vi "WaitForConnection.vi"(8 "error in (no error)":errorcluster, 11 "Tcp in":refnum<class "Tcp.lvclass">) -> (0 "error out":errorcluster, 3 "Tcp out":refnum<class "Tcp.lvclass">)   [LabVIEW 2022 SP3, in "Tcp.lvlib" / "Tcp.lvclass"]
uses:
  Tcp.lvclass
  Tcp.lvclass/Tcp.ctl
  <vilib>/ActorFramework/Actor/Actor.lvclass
  Connection/Connection/Connection.lvclass
  Connection/Connection Messages/Initialize Msg/Initialize Msg.lvclass
  C:/Program Files (x86)/National Instruments/LabVIEW 2022/vi.lib/ActorFramework/Actor/Actor.lvclass
  Tcp Messages/WaitForConnection Msg/WaitForConnection Msg.lvclass
  TcpSocket/Source/TcpSocket/TcpServer/TcpServer.lvclass
  TcpSocket/Source/TcpSocket/Connection/Connection.lvclass
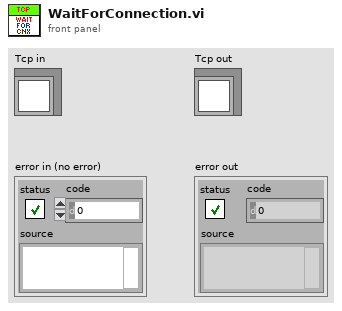
[diagram p1: front panel]
types:
  T1 = map{u64, refnum<class "Message Enqueuer.lvclass">}
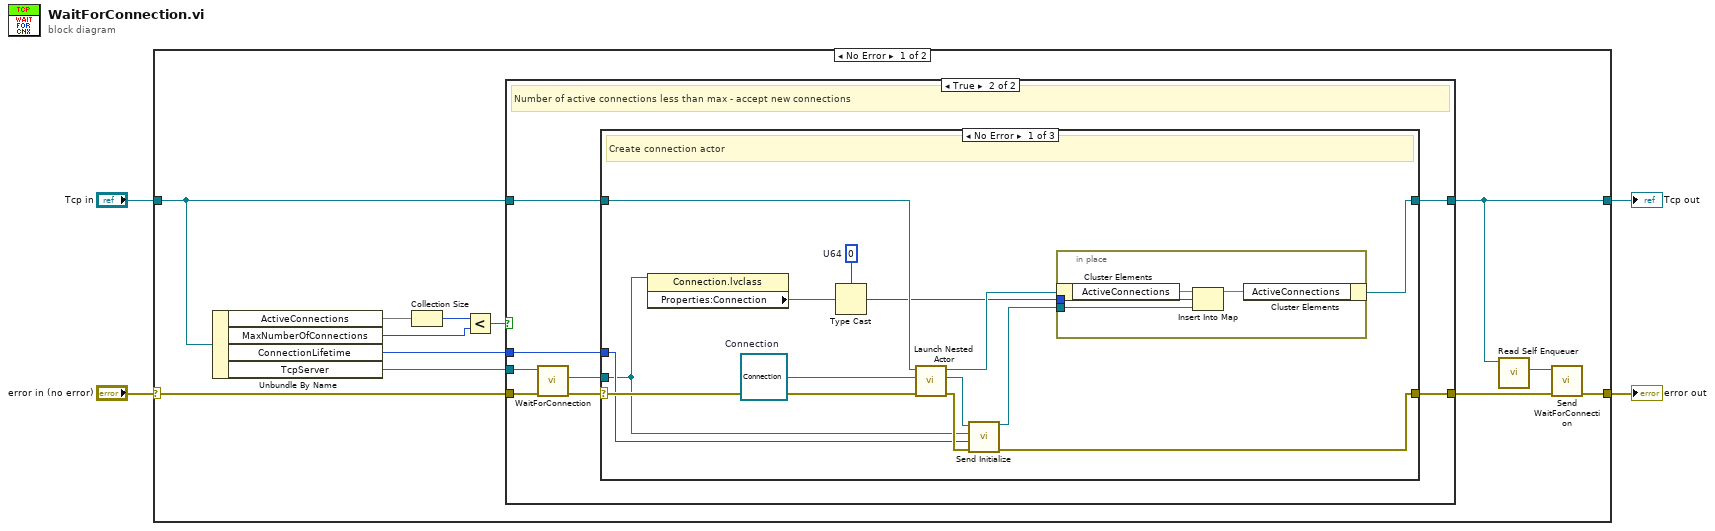
[diagram p0: block diagram]
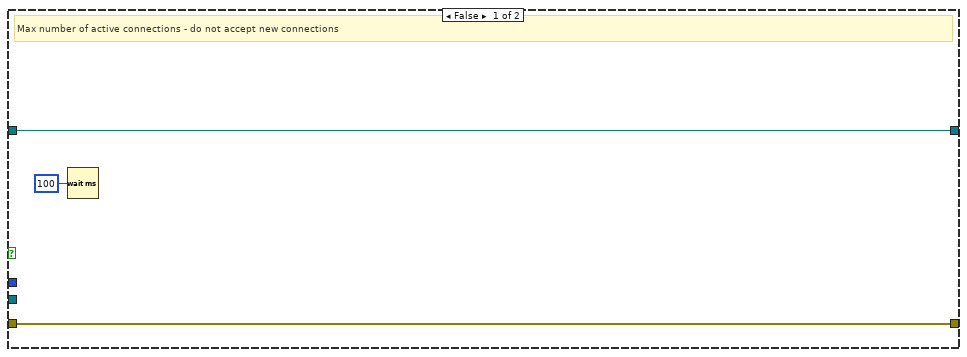
[diagram p2: hidden frame]
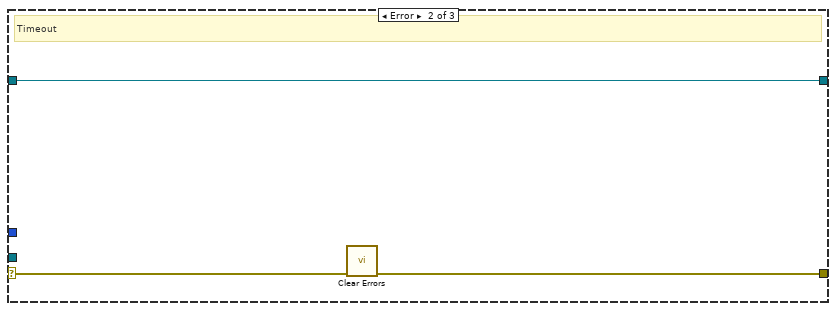
[diagram p3: hidden frame]
diagram:
  n1 = case shown="No Error" "error in (no error)" {
    selector: "error in (no error)" -> [w16 w52]
    tunnel: [w10 w52] -> w3
    tunnel: [w12 w51] -> w1
    tunnel: "Tcp in" -> [w14 w51]
    frame No Error {
      n2 = Unbundle By Name(w14) -> ("ActiveConnections"=w8:T1, "MaxNumberOfConnections"=w6:i32, "ConnectionLifetime"=w13:i32, "TcpServer"=w15:refnum<class "TcpServer.lvclass">)
      n3 = Collection Size(1:w8) -> (0:w7:i32)
      n4 = Less?(x=w7, y=w6) -> (x < y?=w5:bool)
      n5 = case shown="True" w5 {
        tunnel: w16 -> [w19 w27]
        tunnel: w15 -> [_ w24]
        tunnel: w14 -> [w18 w23]
        tunnel: w13 -> [_ w22]
        tunnel: [w18 w21] -> w12
        tunnel: [w19 w20] -> w11
        frame False {
          # "Max number of active connections - do not accept new connections"
          n6 = Wait (ms)(milliseconds to wait=u32 100) -> ()  [unwired: 1 out]
        }
        frame True {
          # "Number of active connections less than max - accept new connections"
          n7 = call-dynamic "WaitForConnection.vi"("error in (no error)"=w27, "TcpServer in"=w24) -> ("error out"=w26:errorcluster, "Connection"=w25:refnum<class "Connection.lvclass">)  [unwired: 7 in, 1 out]
          n8 = case shown="No Error" w26 {
            selector: w26 -> [w41 w48 w50]
            tunnel: [w35 w46 w50] -> w20
            tunnel: w25 -> [w31 _ _]
            tunnel: w23 -> [w39 w47 w49]
            tunnel: [w32 w47 w49] -> w21
            tunnel: w22 -> [w36 _ _]
            frame No Error {
              w28 = u64 0  # U64
              w40 = refnum<class "Connection.lvclass"> refnum  # Connection
              # "Create connection actor"
              n9 = property class="Connection.lvclass"(reference=w31) -> ("Properties:Connection"=w30:refnum<k5>)  [unwired: 1 in, 2 out]
              n10 = Type Cast(type=w28, x=w30) -> (*(type *) &x=w29:u64)
              n11 = call <vilib>:"Launch Nested Actor.vi"("error in (no error)"=w41, "Nested Actor"=w40, "Caller Actor in"=w39) -> ("error out"=w37:errorcluster, "Nested Actor's Enqueuer"=w38:refnum<class "Message Enqueuer.lvclass">, "Caller Actor out"=w33:refnum<class "Tcp.lvclass">)  [unwired: 6 in]
              n12 = call "Send Initialize.vi"("error in (no error)"=w37, "Timeout [ms] (5000)"=w36, "Connection"=w31, "Message Enqueuer"=w38) -> ("error out"=w35:errorcluster, "Message Enqueuer out"=w34:refnum<class "Message Enqueuer.lvclass">)  [unwired: 6 in]
              n13 = in-place {
                in-place-border: w34 -> [w43]
                in-place-border: w29 -> [w42]
                n14 = in-place-cluster #1(w33) -> ("ActiveConnections"=w45:T1)
                n15 = Insert Into Map(map in=w45, key=w42, value=w43) -> (map out=w44:T1)  [unwired: 2 out]
                n16 = in-place-cluster #1("ActiveConnections"=w44) -> (w32:refnum<class "Tcp.lvclass">)
              }
            }
            frame Error {
              # "Timeout"
              n17 = call <vilib>:"Clear Errors.vi"("error in (no error)"=w48) -> ("error out"=w46:errorcluster)  [unwired: 5 in, 1 out]
            }
            frame Default {
              # "Error"
            }
          }
        }
      }
      n18 = call <vilib>:"Read Self Enqueuer.vi"("Actor"=w12) -> ("Self Enqueuer"=w9:refnum<class "Message Enqueuer.lvclass">)  [unwired: 10 in]
      n19 = call "Send WaitForConnection.vi"("error in (no error)"=w11, "Message Enqueuer"=w9) -> ("error out"=w10:errorcluster)  [unwired: 8 in, 1 out]
    }
    frame Error {
    }
  }
  "error out" <- w3
  "Tcp out" <- w1
